vi "Encoder_sub_VI.vi"(8 "error in (no error)":errorcluster, 11 "Encoder Input":T2) -> (0 "error out":errorcluster, 3 "Encoder Output":T2)   [LabVIEW 2017]
uses:
  <vilib>/myRIO/Common/Instrument Driver Framework/myRIO v1.0/Encoder/typedefs/Encoder Count Direction Enum.ctl
  <vilib>/myRIO/Common/Instrument Driver Framework/myRIO v1.0/Encoder/typedefs/Encoder Signal Mode.ctl
  <vilib>/myRIO/Common/Instrument Driver Framework/myRIO v1.0/Encoder/typedefs/Encoder Channels Enum.ctl
  <vilib>/myRIO/Common/Instrument Driver Framework/Utilities/typedefs/Generic FPGA Reference.ctl
  <vilib>/myRIO/Common/Instrument Driver Framework/Utilities/typedefs/myRIO v1.0 Reference.ctl
  <vilib>/myRIO/Common/Instrument Driver Framework/Utilities/typedefs/Hardware Version Enum.ctl
  <vilib>/myRIO/Common/Instrument Driver Framework/Utilities/typedefs/myRIO Generic Hardware Reference.ctl
  <vilib>/myRIO/Instrument Drivers/Onboard IO/Encoder/typedefs/Encoder Reference.ctl
  <vilib>/myRIO/Instrument Drivers/Onboard IO/Encoder/Encoder.lvlib
  <vilib>/myRIO/Instrument Drivers/Onboard IO/Encoder/vis/Read.vi
  <vilib>/myRIO/Common/Instrument Driver Framework/myRIO v1.0/Encoder/typedefs/Encoder Configuration v1.0.ctl
  <vilib>/userdefined/High Color/nirio_resource_hc.ctl
  <vilib>/myRIO/Common/Instrument Driver Framework/myRIO v1.0/Encoder/vis/myRIO v1.1 Open Encoder.vi
  <vilib>/myRIO/Common/Instrument Driver Framework/myRIO v1.0/Encoder/vis/myRIO v1.0 Configure Encoder.vi
  <vilib>/myRIO/Instrument Drivers/Onboard IO/Encoder/vis/myRIO Encoder Open.xnode
  <vilib>/myRIO/Common/Instrument Driver Framework/Utilities/vis/Is FPGA Ref Available.vi
  <vilib>/myRIO/Express VI/Onboard IO/Encoder/Encoder Express VI.xnode
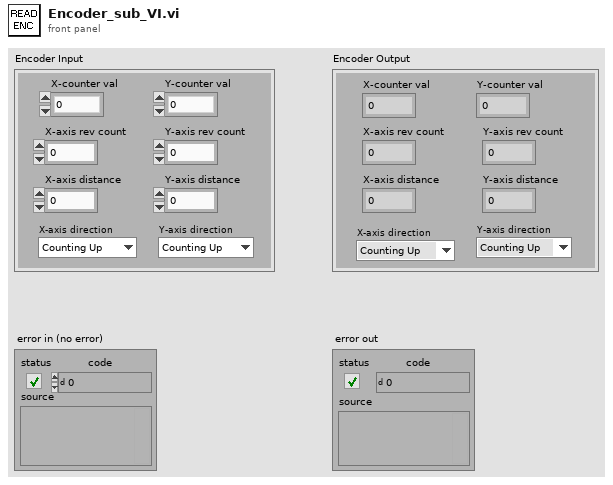
[diagram p1: front panel]
types:
  T1 = typedef "Encoder Count Direction Enum.ctl" = enum16{"Counting Up", "Counting Down"}
  T2 = cluster{"Y-axis rev count":dbl, "Y-axis distance":dbl, "X-axis rev count":dbl, "X-axis distance":dbl, "Y-axis direction":T1, "X-axis direction":T1, "X-counter val":i32, "Y-counter val":i32}
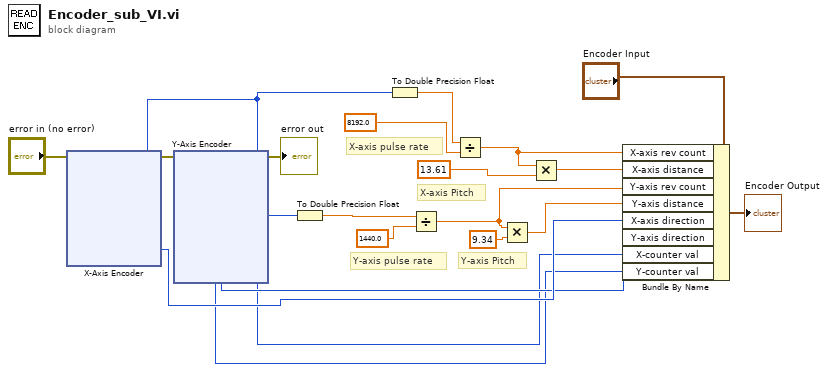
[diagram p0: block diagram]
diagram:
  # "Y-axis Pitch"
  # "Y-axis pulse rate"
  # "X-axis pulse rate"
  # "X-axis Pitch"
  n1 = xnode "X-Axis Encoder"("error in (no error)"="error in (no error)") -> ("Counter Value"=w4:i32, "Counter Direction"=w7:T1, "error out"=w16:errorcluster)  [unwired: 1 in, 1 out]
  n2 = xnode "Y-Axis Encoder"("error in (no error)"=w16) -> ("Counter Value"=w5:i32, "Counter Direction"=w6:T1, "error out"=→"error out":errorcluster)  [unwired: 1 in, 1 out]
  n3 = To Double Precision Float(number=w5) -> (double precision float=w3:dbl)
  n4 = To Double Precision Float(number=w4) -> (double precision float=w2:dbl)
  n5 = Divide(x=w3, y=1440.0) -> (x/y=w11:dbl)
  n6 = Divide(x=w2, y=8192.0) -> (x/y=w1:dbl)
  n7 = Multiply(x=w11, y=9.34) -> (x*y=w14:dbl)
  n8 = Multiply(x=w1, y=13.61) -> (x*y=w15:dbl)
  n9 = Bundle By Name(cluster="Encoder Input", "X-axis rev count"=w1, "X-axis distance"=w15, "Y-axis rev count"=w11, "Y-axis distance"=w14, "X-axis direction"=w7, "Y-axis direction"=w6, "X-counter val"=w4, "Y-counter val"=w5) -> (→"Encoder Output":T2)
